vi "M808placer.vi"(0 "Gcode Array in":string[](array[string]), 5 "Line # start":u32, 7 "Line # end":u32, 9 "Gcode line # array in":i32[](array[numeric]), 11 "error in":errorcluster, 12 "Loop count":u32) -> (4 "Gcode Array out":string[](array[string]), 15 "error out":errorcluster)   [LabVIEW 2020]
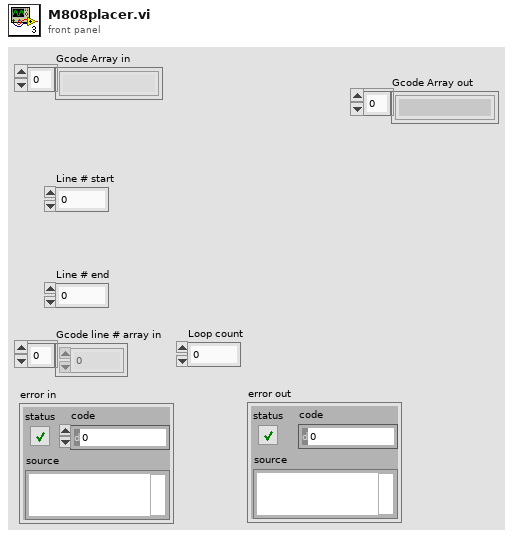
[diagram p1: front panel]
types:
  T1 = enum16{"open", "replace", "create", "open or create", "replace or create", "replace or create with confirmation"}
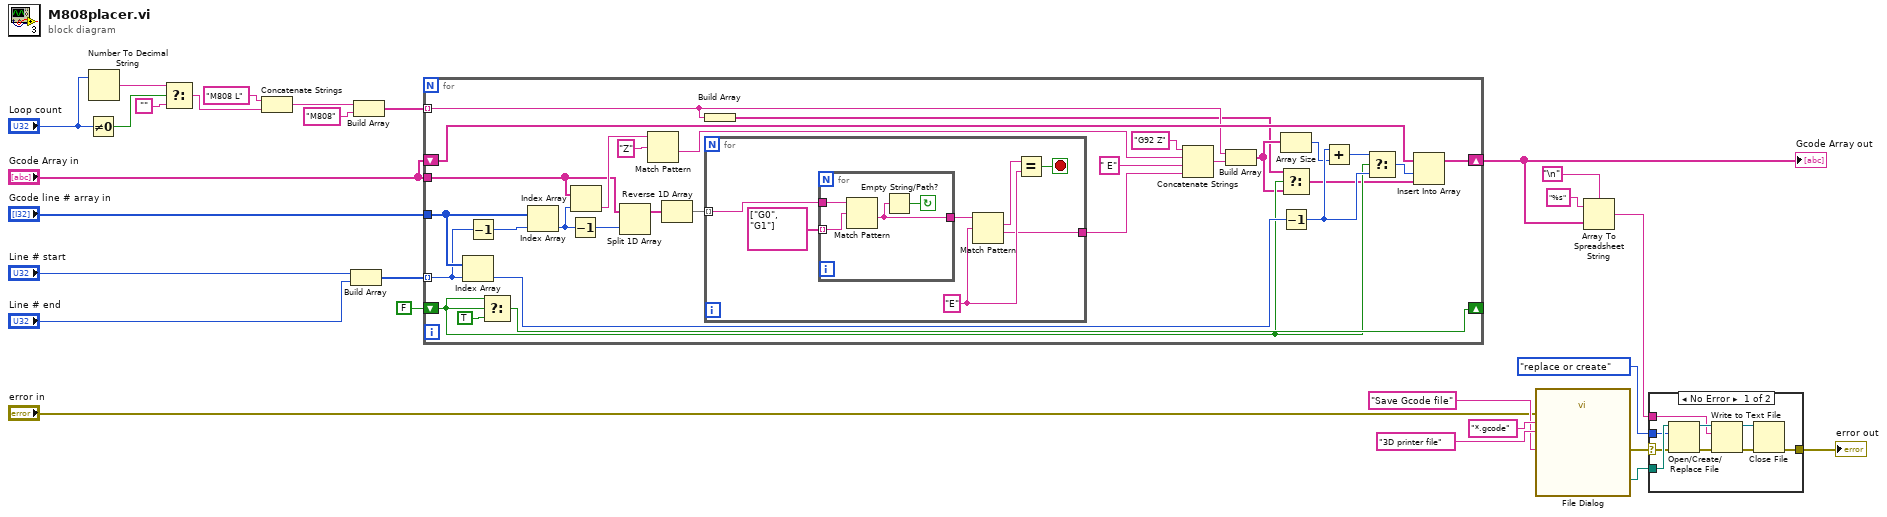
[diagram p0: block diagram]
diagram:
  n1 = Not Equal To 0?(x="Loop count") -> (x != 0?=w16:bool)
  n2 = Number To Decimal String(number="Loop count") -> (decimal integer string=w15:string)  [unwired: 1 in]
  n3 = Select(t=w15, s=w16, f="") -> (s? t:f=w14:string)
  n4 = Concatenate Strings("M808 L" ("string"), w14) -> (w21:string)
  n5 = Build Array("Line # start", "Line # end") -> (w24:u32[])
  n6 = Build Array(w21, "M808" ("element")) -> (w25:string[])
  n7 = for {
    tunnel: "Gcode line # array in" -> [w44]
    tunnel: "Gcode Array in" -> [w42]
    tunnel: w25 -> [w29] mode=indexing
    tunnel: w24 -> [w41] mode=indexing
    shift-right: [w39] -> w12
    shift-left: "Gcode Array in" -> [w40]
    shift-right: [w37] -> _
    shift-left: FALSE -> [w32]
    n8 = Index Array(array=w44, index=w41) -> (element=w43:i32)
    n9 = Decrement(x=w41) -> (x-1=w56:u32)
    n10 = Select(t=w32, s=w32, f=TRUE) -> (s? t:f=w37:bool)
    n11 = Index Array(array=w44, index=w56) -> (element=w52:i32)
    n12 = Decrement(x=w52) -> (x-1=w46:i32)
    n13 = Index Array(array=w42, index=w52) -> (element=w55:string)
    n14 = Split 1D Array(array=w42, index=w46) -> (first subarray=w54:string[])  [unwired: 1 out]
    n15 = Match Pattern(string=w55, regular expression="Z") -> (after substring=w49:string)  [unwired: 1 in, 3 out]
    n16 = Reverse 1D Array(array=w54) -> (reversed array=w53:string[])
    n17 = Build Array(w29) -> (w28:string[])
    n18 = for {
      tunnel: w53 -> [w59] mode=indexing
      tunnel: [w57] -> w47
      stop <- w61 stop-if-true
      w62 = "E" ("regular expression")
      n19 = for {
        tunnel: string[] ["G0", "G1"] ("regular expression") -> [w66] mode=indexing
        tunnel: w59 -> [w67]
        tunnel: [w65] -> w58
        stop <- w64 continue-if-true
        n20 = Match Pattern(string=w67, regular expression=w66) -> (after substring=w65:string)  [unwired: 1 in, 3 out]
        n21 = Empty String/Path?(string/path=w65) -> (empty?=w64:bool)
      }
      n22 = Match Pattern(string=w58, regular expression=w62) -> (match substring=w63:string, after substring=w57:string)  [unwired: 1 in, 2 out]
      n23 = Equal?(x=w63, y=w62) -> (x = y?=w61:bool)
    }
    n24 = Concatenate Strings("G92 Z" ("string"), w49, " E" ("string"), w47) -> (w45:string)
    n25 = Build Array(w29, w45) -> (w31:string[])
    n26 = Array Size(array=w31) -> (size(s)=w34:i32)
    n27 = Select(t=w28, s=w32, f=w31) -> (s? t:f=w30:string[])
    n28 = Decrement(x=w43) -> (x-1=w35:i32)
    n29 = Add(x=w35, y=w34) -> (x+y=w33:i32)
    n30 = Select(t=w33, s=w32, f=w35) -> (s? t:f=w36:i32)
    n31 = Insert Into Array(array=w40, index=w36, new element=w30) -> (w39:string[])
  }
  "Gcode Array out" <- w12
  n32 = call "File Dialog"("prompt"="Save Gcode file", "error in"="error in", "pattern (all files)"="*.gcode", "pattern label"="3D printer file") -> ("selected path"=w9:path, "error out"=w2:errorcluster)  [unwired: 8 in, 2 out]
  n33 = Array To Spreadsheet String(delimiter (Tab)="\n", array=w12, 3:"%s" ("format string")) -> (spreadsheet string=w4:string)
  n34 = case shown="No Error" w2 {
    selector: w2 -> [w68 _]
    tunnel: w9 -> [w76 _]
    tunnel: T1."replace or create" ("operation (0:open)") -> [w75 _]
    tunnel: w4 -> [w72 _]
    tunnel: [w69 _] -> w3
    frame No Error {
      n35 = Open/Create/Replace File(file path (use dialog)=w76, error in=w68, operation (0:open)=w75) -> (refnum out=w74:refnum<file>, error out=w73:errorcluster)  [unwired: 3 in, 1 out]
      n36 = Write to Text File(file (use dialog)=w74, text=w72, error in=w73) -> (refnum out=w71:refnum<file>, error out=w70:errorcluster)  [unwired: 1 in, 1 out]
      n37 = Close File(refnum=w71, error in=w70) -> (error out=w69:errorcluster)  [unwired: 1 out]
    }
    frame Error {
    }
  }
  "error out" <- w3
